vi "固件升级对话框.vi"() -> ()   [LabVIEW 2016, in "斯坦道总氮.lvlib"]
uses:
  <vilib>/Utility/miscctls.llb/LVPointTypeDef.ctl
panel:
  in  "关闭":bool
  in  "固件升级":bool
  in  "固件状态":bool
  out "结果字符串":string
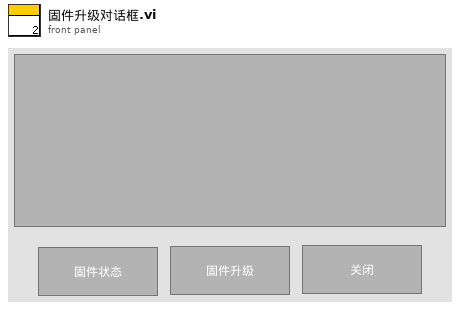
[diagram p1: front panel]
types:
  T1 = typedef "LVPointTypeDef.ctl" = cluster{"Horizontal":i16, "Vertical":i16}
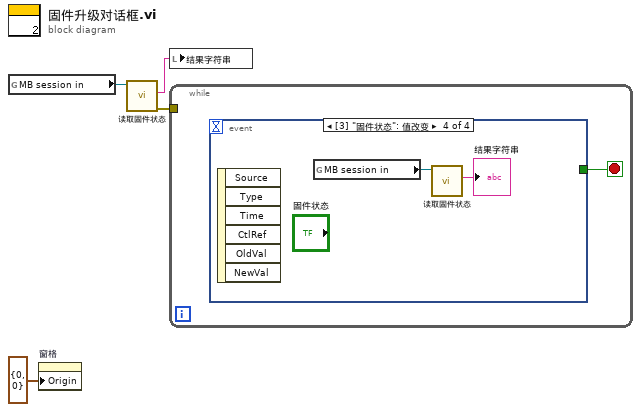
[diagram p0: block diagram]
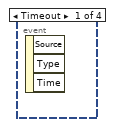
[diagram p2: hidden frame]
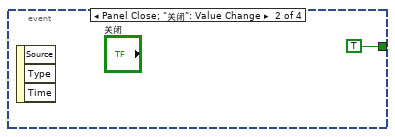
[diagram p3: hidden frame]
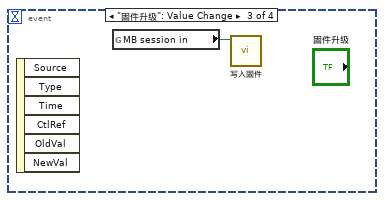
[diagram p4: hidden frame]
diagram:
  n1 = global read "VAR总氮全局变量.vi" "MB session in"() -> (w3:refnum<class "MB_Master.lvclass">)
  n2 = property on="窗格" class="Pane"("Origin"=T1 {"Horizontal"=0, "Vertical"=0} ("原点")) -> ()  [unwired: 2 in, 2 out]
  n3 = call "读取固件状态.vi"("MB session in"=w3) -> ("error out"=w1:errorcluster, "结果字符串"=w2:string)  [unwired: 8 in, 1 out]
  n4 = local write "结果字符串"(w2) -> ()
  n5 = while {
    tunnel: w1 -> [_]
    stop <- w5 stop-if-true
    n6 = event shown="[3] \"固件状态\": 值改变" {
      selector: _ -> [_ _ _ _]
      dyn-events: _ -> [_ _ _ _]
      timeout: _ -> [_ _ _ _]
      tunnel: [_ TRUE _ _] -> w5
      event Timeout {
        n7 = event-data() -> ()  [unwired: 1 in, 3 out]
      }
      event Panel Close; "关闭": Value Change {
        n8 = event-data() -> ()  [unwired: 1 in, 3 out]
      }
      event "固件升级": Value Change {
        n9 = event-data() -> ()  [unwired: 1 in, 6 out]
        n10 = global read "VAR总氮全局变量.vi" "MB session in"() -> (w7:refnum<class "MB_Master.lvclass">)
        n11 = call "写入固件.vi"("MB session in"=w7) -> ()  [unwired: 9 in, 2 out]
      }
      event "固件状态": Value Change {
        n12 = event-data() -> ()  [unwired: 1 in, 6 out]
        n13 = global read "VAR总氮全局变量.vi" "MB session in"() -> (w8:refnum<class "MB_Master.lvclass">)
        n14 = call "读取固件状态.vi"("MB session in"=w8) -> ("结果字符串"=→"结果字符串":string)  [unwired: 8 in, 2 out]
      }
    }
  }
